vi "Collect Components UI.vi"(8 "error in (no error)":errorcluster, 10 "User Interface Handler":refnum<class "User Interface Handler.lvclass">, 11 "Item Ref in":T2 format="%.0x") -> (0 "error out":errorcluster, 2 "component settings":T1[](array[typedef]), 3 "Item Ref out":T2=18446744073709551615 format="%.0x")   [LabVIEW 2017, in "DSF System Explorer.lvlib"]
uses:
  DSF System Explorer.lvlib
  <vilib>/NI Veristand/Custom Device API/Custom Device Item Ref.ctl
  DSF Core.lvlibp/Classes/User Interface Handler/User Interface Handler.lvclass
  DSF Core.lvlibp/Typedefs/DSF Settings Info.ctl
  DSF Core.lvlibp/Classes/User Interface/Plugin/Component Settings Editor.lvclass
  <vilib>/NI Veristand/Custom Device API/Custom Device API.lvlib
  DSF Core.lvlibp
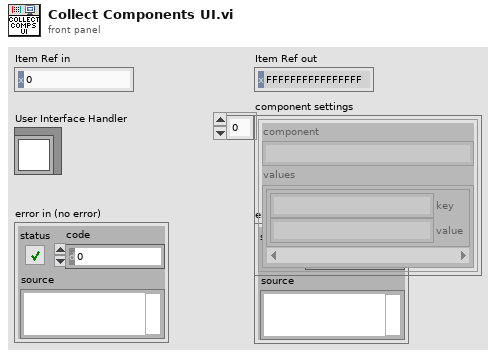
[diagram p1: front panel]
types:
  T1 = typedef "DSF Core.lvlibp/DSF Settings Info.ctl" = cluster{"component":string, "values":cluster{"key":string, "value":string}[]}
  T2 = typedef "Custom Device API.lvlib/Custom Device Item Ref.ctl" = u64
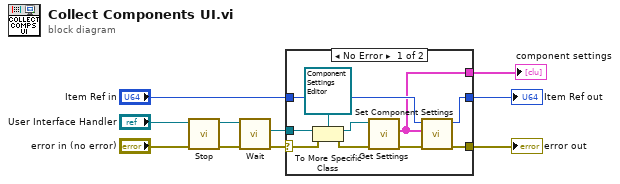
[diagram p0: block diagram]
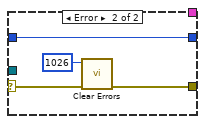
[diagram p2: hidden frame]
diagram:
  n1 = call "Stop.vi"("error in (no error)"="error in (no error)", "User Interface Handler in"="User Interface Handler") -> ("error out"=w4:errorcluster, "User Interface Handler out"=w5:refnum<class "User Interface Handler.lvclass">)  [unwired: 8 in]
  n2 = call "Wait.vi"("error in (no error)"=w4, "User Interface Handler in"=w5) -> ("error out"=w7:errorcluster, "User Interface"=w8:refnum<class "User Interface.lvclass">)  [unwired: 7 in, 1 out]
  n3 = case shown="No Error" w7 {
    selector: w7 -> [w17 w23]
    tunnel: w8 -> [w18 _]
    tunnel: "Item Ref in" -> [w15 w21]
    tunnel: [w20 w22] -> w10
    tunnel: [w12 w21] -> w2
    tunnel: [w11 _] -> w1
    frame No Error {
      n4 = To More Specific Class(target class=refnum<class "Component Settings Editor.lvclass"> refnum ("Component Settings Editor in"), reference=w18, error in=w17) -> (specific class reference=w13:refnum<class "Component Settings Editor.lvclass">, error out=w16:errorcluster)
      n5 = call "Get Settings.vi"("error in (no error)"=w16, "Component Settings Editor in"=w13) -> ("error out"=w19:errorcluster, "component settings"=w11:T1[])  [unwired: 7 in, 1 out]
      n6 = call "Set Component Settings.vi"("error in (no error)"=w19, "component settings"=w11, "Item Ref in"=w15) -> ("error out"=w20:errorcluster, "Item Ref out"=w12:T2)  [unwired: 7 in]
    }
    frame Error {
      n7 = call <vilib>:"Clear Errors.vi"("error in (no error)"=w23, "specific error code to clear (0: all)"=1026) -> ("error out"=w22:errorcluster)  [unwired: 4 in, 1 out]
    }
  }
  "error out" <- w10
  "Item Ref out" <- w2
  "component settings" <- w1
